vi "Facade.vi"(0 "Data In":T4, 2 "Display State In":T2, 3 "Container State":T3) -> (6 "Data Out":T4, 7 "Display State Out":T2, 8 "Action":T1)   [LabVIEW 2020, in "KLegend.xctl"]
uses:
  KLegend.xctl
  Data.vi
  <vilib>/_xctls/Container State.ctl
  State.vi
  <vilib>/_xctls/Action.ctl
  <vilib>/_xctls/XControlSupport.lvlib
panel:
  in  "Listbox":i32(listbox)
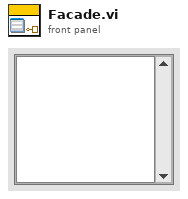
[diagram p1: front panel]
types:
  T1 = typedef "XControlSupport.lvlib/Action.ctl" = cluster{"Data Changed?":bool, "State Changed?":bool, "Action Name":string}
  T2 = typedef "KLegend.xctl/State.vi" = cluster{"Plot":refnum<vi>, "Vals":dbl[], "fmt":string, "cmd":string, "max rows":i32}
  T3 = typedef "XControlSupport.lvlib/Container State.ctl" = cluster{"Indicator?":bool, "Run Mode?":bool, " Refnum":refnum<vi>}
  T4 = typedef "KLegend.xctl/Data.vi" = dbl
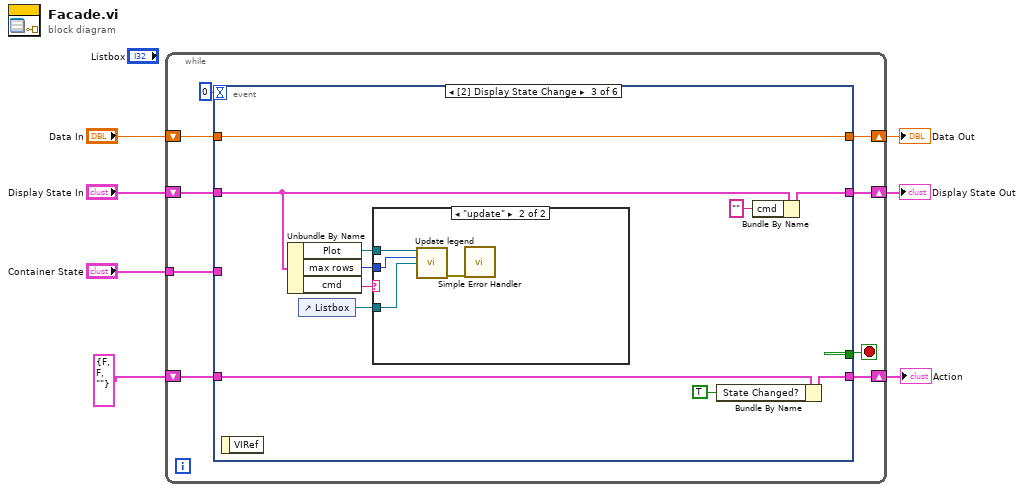
[diagram p0: block diagram]
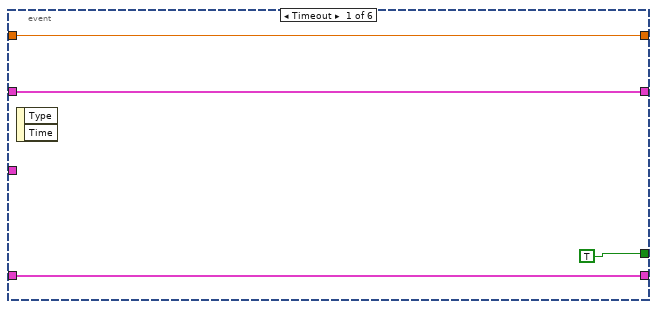
[diagram p2: hidden frame]
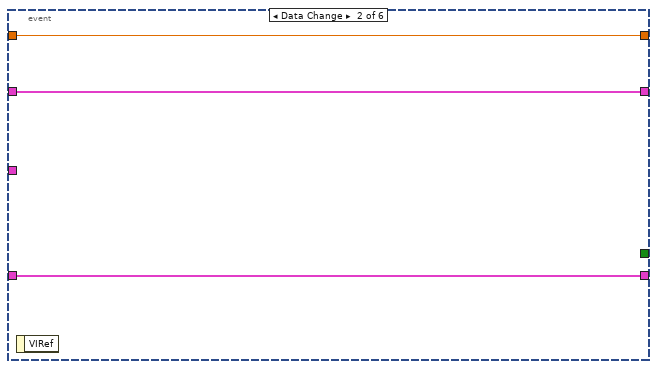
[diagram p3: hidden frame]
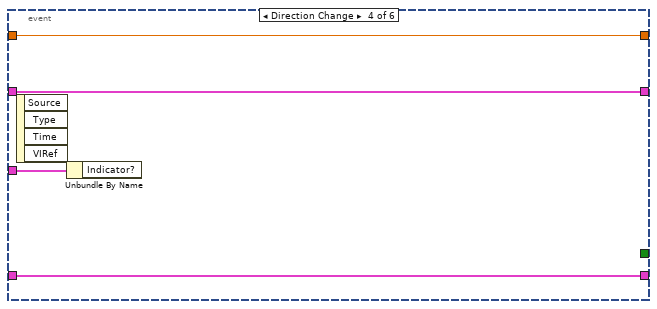
[diagram p5: hidden frame]
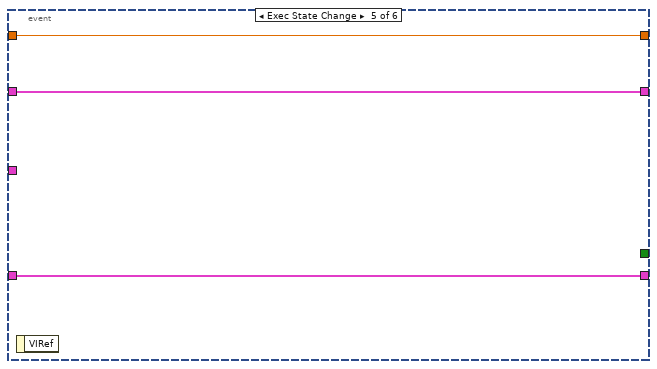
[diagram p6: hidden frame]
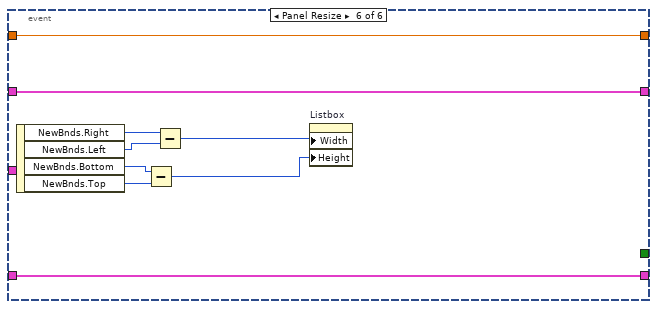
[diagram p7: hidden frame]
diagram:
  n1 = while {
    shift-right: [w15] -> w4
    shift-left: "Display State In" -> [w16]
    tunnel: "Container State" -> [w12]
    shift-right: [w10] -> w7
    shift-left: "Data In" -> [w11]
    shift-right: [w8] -> w2
    shift-left: T1 {"Data Changed?"=FALSE, "State Changed?"=FALSE, "Action Name"=""} ("Action") -> [w9]
    stop <- w14 stop-if-true
    n2 = event shown="[2] Display State Change" {
      selector: _ -> [_ _ _ _ _ _]
      dyn-events: _ -> [_ _ _ _ _ _]
      timeout: 0 -> [_ _ _ _ _ _]
      tunnel: w16 -> [w18 w22 w32 w41 w45 w54]
      tunnel: [w18 w22 w29 w41 w45 w54] -> w15
      tunnel: [TRUE _ _ _ _ _] -> w14
      tunnel: w12 -> [_ _ _ w42 _ _]
      tunnel: w11 -> [w17 w23 w34 w40 w44 w53]
      tunnel: [w17 w23 w34 w40 w44 w53] -> w10
      tunnel: [w19 w21 w31 w39 w43 w52] -> w8
      tunnel: w9 -> [w19 w21 w33 w39 w43 w52]
      event Timeout {
        n3 = event-data() -> ()  [unwired: 1 in, 2 out]
      }
      event Data Change {
        n4 = event-data() -> ()  [unwired: 1 in, 1 out]
      }
      event Display State Change {
        n5 = event-data() -> ()  [unwired: 1 in, 1 out]
        n6 = Unbundle By Name(w32) -> ("Plot"=w27:refnum<vi>, "max rows"=w24:i32, "cmd"=w26:string)
        n7 = control-ref of="Listbox"() -> (w25:refnum<vi>)
        n8 = case shown="\"update\"" w26 {
          tunnel: w27 -> [_ w38]
          tunnel: w25 -> [_ w37]
          tunnel: w24 -> [_ w35]
          frame "", Default {
          }
          frame "update" {
            n9 = call "Update legend.vi"("XYGraph in"=w38, "max rows"=w35, "Listbox"=w37) -> ("error out"=w36:errorcluster)  [unwired: 12 in]
            n10 = call <vilib>:"Simple Error Handler.vi"("error in (no error)"=w36) -> ()  [unwired: 4 in, 5 out]
          }
        }
        n11 = Bundle By Name(cluster=w33, "State Changed?"=TRUE) -> (w31:T1)
        n12 = Bundle By Name(cluster=w32, "cmd"="") -> (w29:T2)
      }
      event Direction Change {
        n13 = event-data() -> ()  [unwired: 1 in, 4 out]
        n14 = Unbundle By Name(w42) -> ()  [unwired: 1 out]
      }
      event Exec State Change {
        n15 = event-data() -> ()  [unwired: 1 in, 1 out]
      }
      event Panel Resize {
        n16 = event-data() -> ("NewBnds.Right"=w51:i16, "NewBnds.Left"=w50:i16, "NewBnds.Bottom"=w48:i16, "NewBnds.Top"=w49:i16)  [unwired: 1 in]
        n17 = Subtract(x=w48, y=w49) -> (x-y=w46:i16)
        n18 = Subtract(x=w51, y=w50) -> (x-y=w47:i16)
        n19 = property on="Listbox" class="LstBox (strict)"("Width"=w47, "Height"=w46) -> ()  [unwired: 2 in, 2 out]
      }
    }
  }
  "Display State Out" <- w4
  "Data Out" <- w7
  "Action" <- w2
